vi "plot1.vi"(8 "error in (no error)":errorcluster, 11 "Counter in":refnum<class "Counter.lvclass">) -> (0 "error out":errorcluster, 3 "Counter out":refnum<class "Counter.lvclass">)   [LabVIEW 2013, in "Counter.lvclass"]
uses:
  Counter.lvclass
  Counter.lvclass/Counter.ctl
panel:
  out "Counters Chart 3":u32[][](graph)
  out "counter data":u32[][](array[numeric])
  out "Counters Chart":u32[][](graph)
  out "current counter totals":u32[](array[numeric])
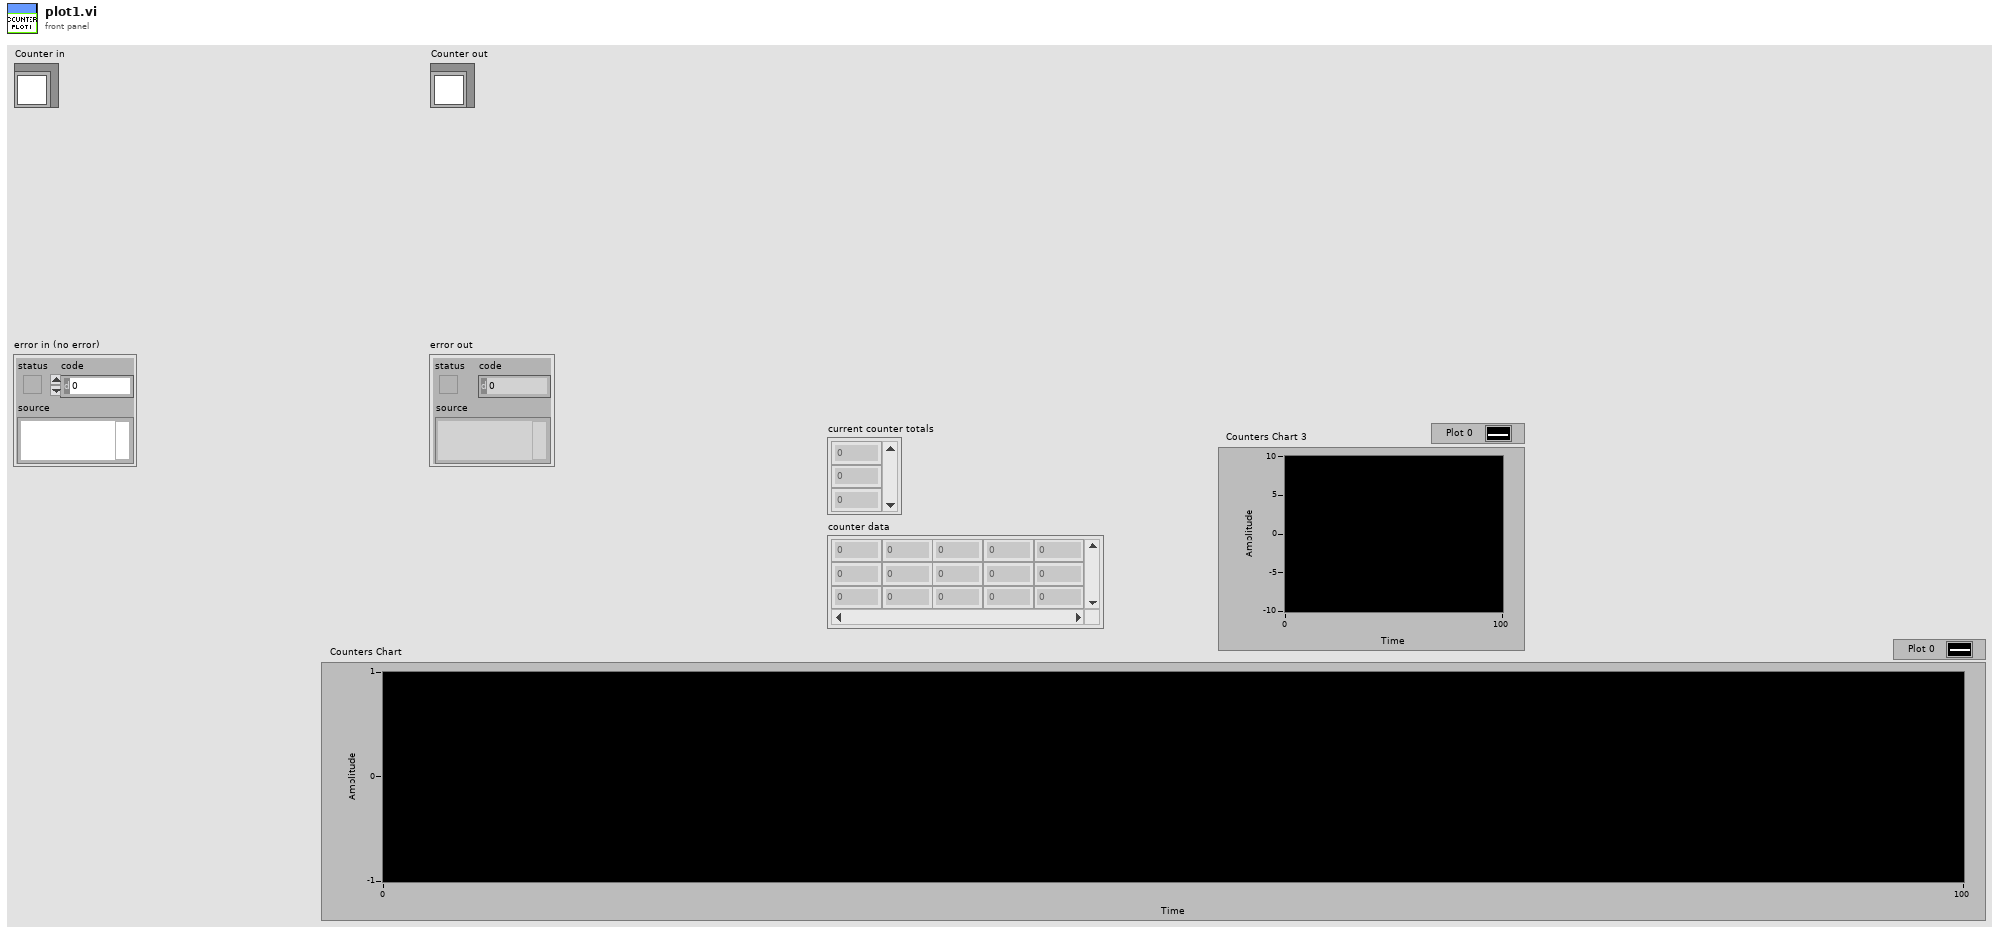
[diagram p1: front panel]
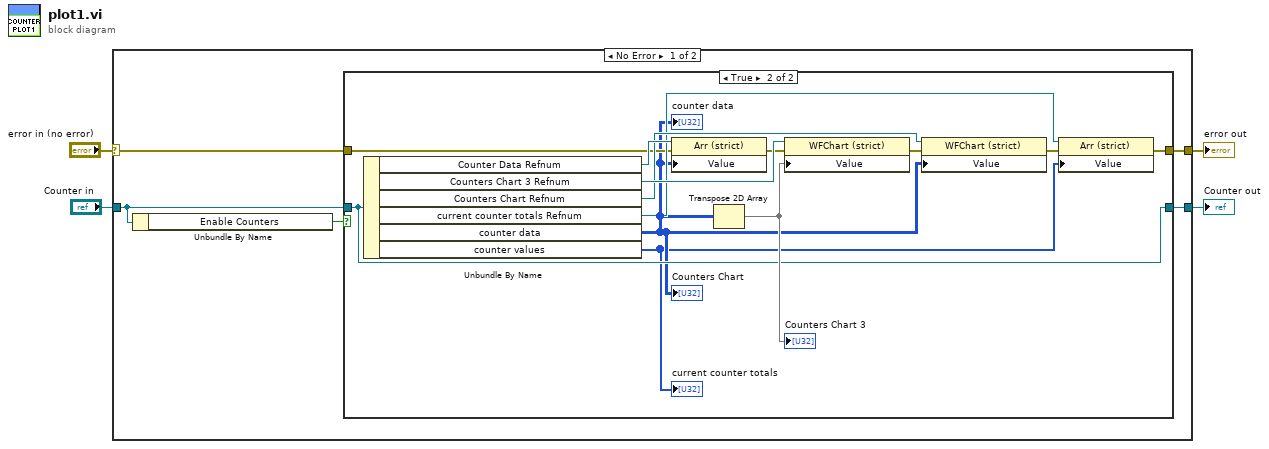
[diagram p0: block diagram]
diagram:
  n1 = case shown="No Error" "error in (no error)" {
    selector: "error in (no error)" -> [w9 w26]
    tunnel: [w8 w26] -> w3
    tunnel: "Counter in" -> [w7 w25]
    tunnel: [w5 w25] -> w1
    frame No Error {
      n2 = Unbundle By Name(w7) -> ("Enable Counters"=w6:bool)
      n3 = case shown="True" w6 {
        tunnel: w9 -> [w10 w16]
        tunnel: [w10 w15] -> w8
        tunnel: w7 -> [w11 w14]
        tunnel: [w11 w14] -> w5
        frame False {
        }
        frame True {
          n4 = Unbundle By Name(w14) -> ("Counter Data Refnum"=w24:refnum<vi>, "Counters Chart 3 Refnum"=w23:refnum<vi>, "Counters Chart Refnum"=w22:refnum<vi>, "current counter totals Refnum"=w21:refnum<vi>, "counter data"=w13:u32[][], "counter values"=w12:u32[])
          "current counter totals" <- w12
          "Counters Chart" <- w13
          "counter data" <- w13
          n5 = property class="Arr (strict)"(reference=w24, error in=w16, "Value"=w13) -> (error out=w20:errorcluster)  [unwired: 1 out]
          n6 = Transpose 2D Array(2D array=w13) -> (transposed array=w17:u32[][])
          "Counters Chart 3" <- w17
          n7 = property class="WFChart (strict)"(reference=w23, error in=w20, "Value"=w17) -> (error out=w19:errorcluster)  [unwired: 1 out]
          n8 = property class="WFChart (strict)"(reference=w22, error in=w19, "Value"=w13) -> (error out=w18:errorcluster)  [unwired: 1 out]
          n9 = property class="Arr (strict)"(reference=w21, error in=w18, "Value"=w12) -> (error out=w15:errorcluster)  [unwired: 1 out]
        }
      }
    }
    frame Error {
    }
  }
  "error out" <- w3
  "Counter out" <- w1
